vi "Read Part Details_RC.vi"(7 "Part Details in":T2, 8 "error in (no error)":errorcluster, 9 "Rack ID":u8, 10 "Part Name":string="HSG 250F (PS03)", 11 "Output Merged Cluster":variant) -> (0 "error out":errorcluster, 3 "Part Details out":T2)   [LabVIEW 2019, in "Rack Controller.lvclass"]
uses:
  Rack Controller.lvclass
  Controls/Part Details_RC.ctl
panel:
  in  "Pats List":T1
  out "Parts List":T3
  out "Error Message":string
  out "VCluster\n out":variant
  in  "Override file path":path=path "C:/Users/veenaj/Desktop/GTRON/02-11-2018/ZenGage V1.3/Configuration file/Rack Controller Parameters Override.json"
  in  "Default file path":path=path "C:/Users/veenaj/Desktop/GTRON/02-11-2018/ZenGage V1.3/Configuration file/Rack Controller Parameters Default.json"
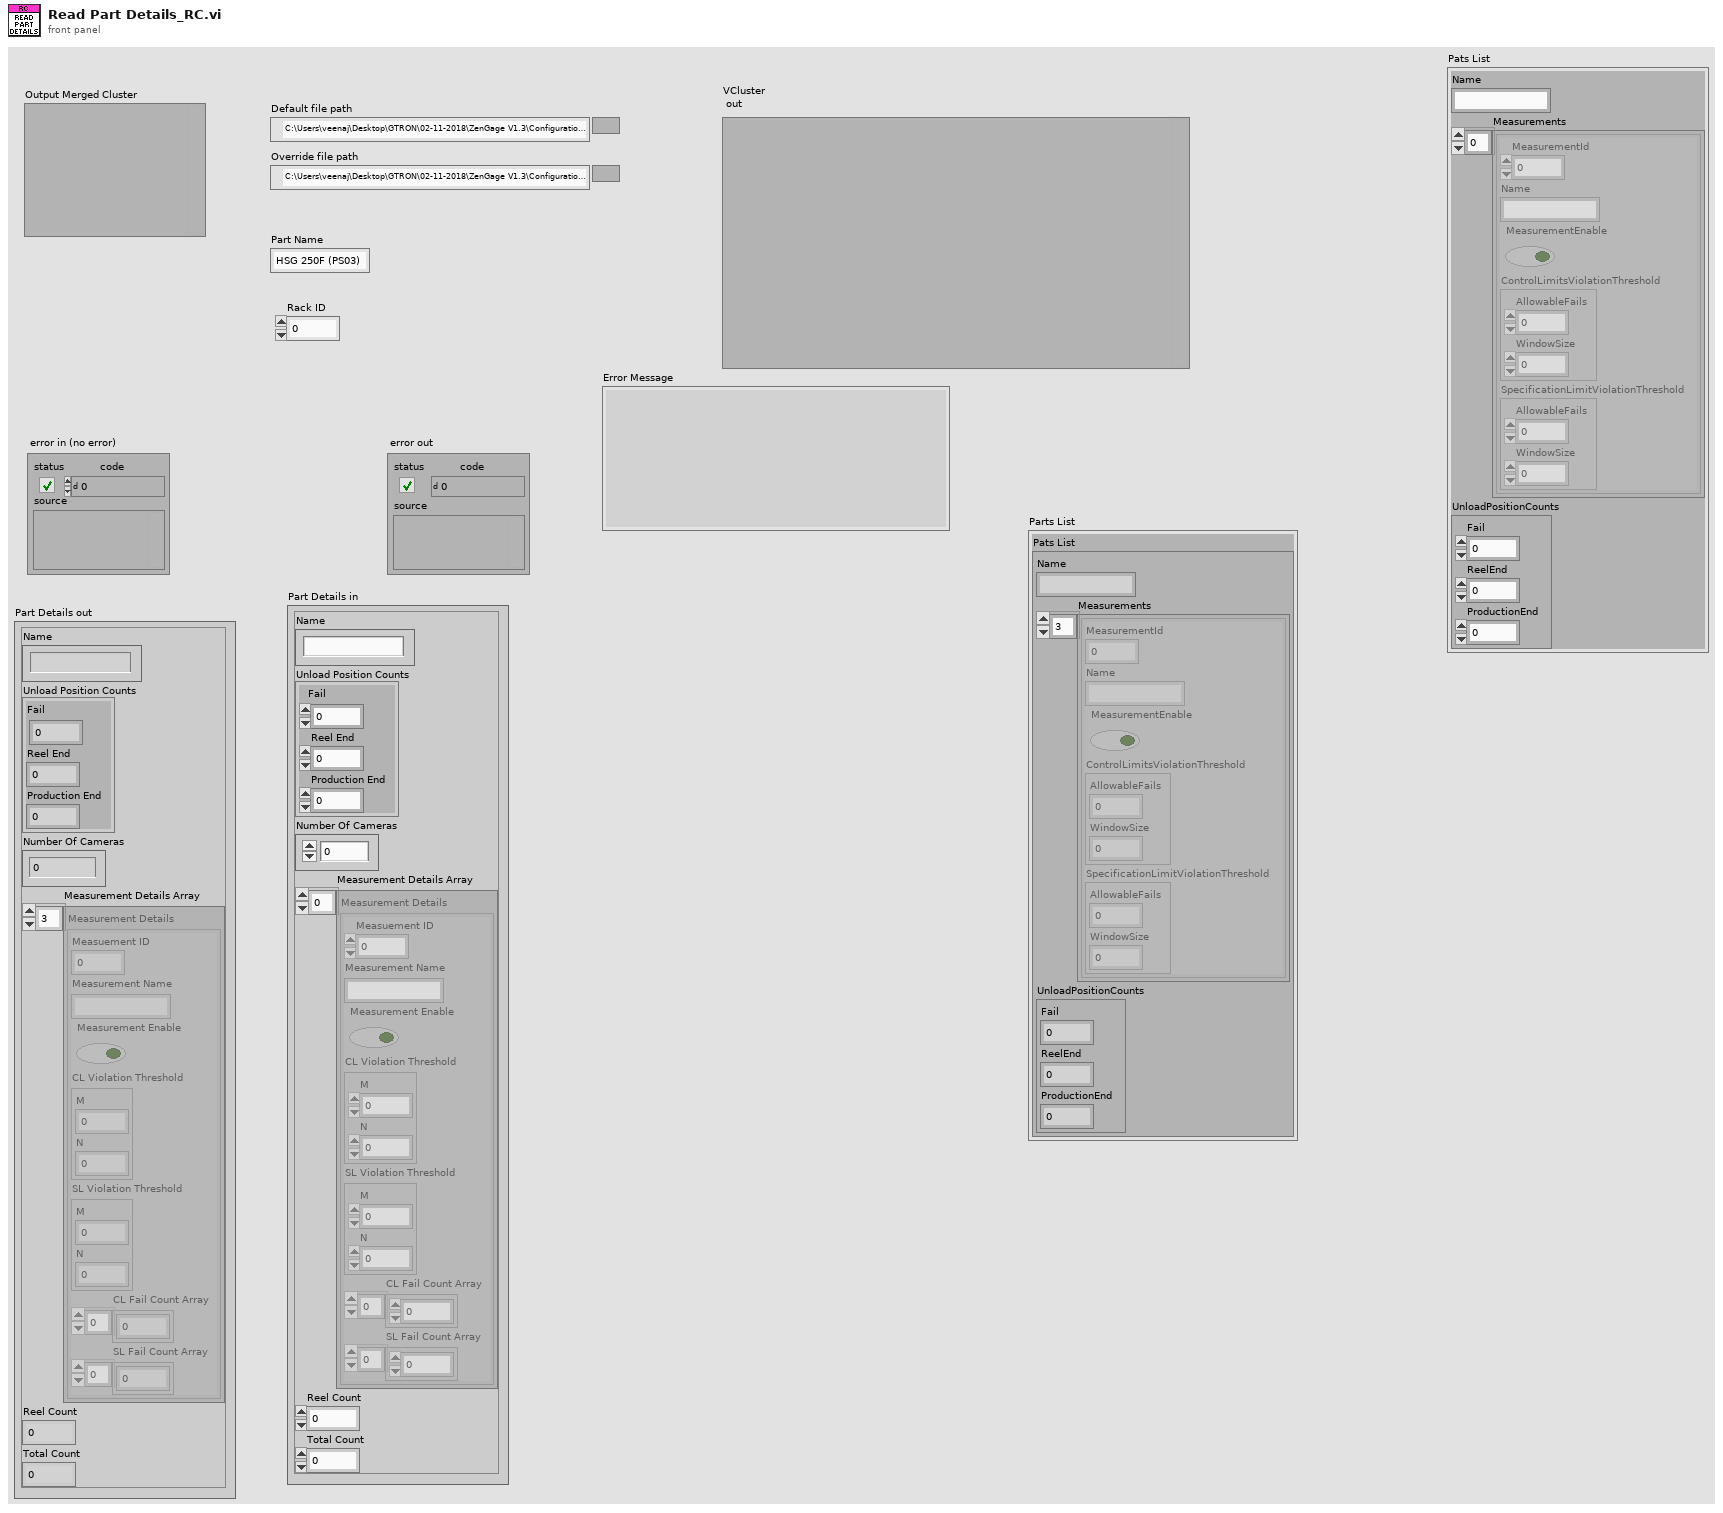
[diagram p1: front panel]
types:
  T1 = cluster{"Name":string, "Measurements":cluster{"MeasurementId":u8, "Name":string, "MeasurementEnable":bool, "ControlLimitsViolationThreshold":cluster{"AllowableFails":u64, "WindowSize":u64}, "SpecificationLimitViolationThreshold":cluster{"AllowableFails":u64, "WindowSize":u64}}[], "UnloadPositionCounts":cluster{"Fail":u64, "ReelEnd":u64, "ProductionEnd":u64}}
  T2 = typedef "Rack Controller.lvclass/Part Details_RC.ctl" = cluster{"Name":string, "Unload Position Counts":cluster{"Fail":u32, "Reel End":u32, "Production End":u32}, "Number Of Cameras":u8, "Measurement Details Array":cluster{"Measuement ID":u16, "Measurement Name":string, "Measurement Enable":bool, "CL Violation Threshold":cluster{"M":u8, "N":u64}, "SL Violation Threshold":cluster{"M":u8, "N":u64}, "CL Fail Count Array":u64[], "SL Fail Count Array":u64[]}[], "Reel Count":u64, "Total Count":u64}
  T3 = cluster{"Pats List":cluster{"Name":string, "Measurements":cluster{"MeasurementId":dbl, "Name":string, "MeasurementEnable":bool, "ControlLimitsViolationThreshold":cluster{"AllowableFails":dbl, "WindowSize":dbl}, "SpecificationLimitViolationThreshold":cluster{"AllowableFails":dbl, "WindowSize":dbl}}[], "UnloadPositionCounts":cluster{"Fail":dbl, "ReelEnd":dbl, "ProductionEnd":dbl}}}
  T4 = cluster{"Pats List":cluster{"Name":string, "Measurements":cluster{"MeasurementId":u8, "Name":string, "MeasurementEnable":bool, "ControlLimitsViolationThreshold":cluster{"AllowableFails":u64, "WindowSize":u64}, "SpecificationLimitViolationThreshold":cluster{"AllowableFails":u64, "WindowSize":u64}}[], "UnloadPositionCounts":cluster{"Fail":u64, "ReelEnd":u64, "ProductionEnd":u64}}}
  T5 = cluster{"Fail":u64, "ReelEnd":u64, "ProductionEnd":u64}
  T6 = cluster{"MeasurementId":u8, "Name":string, "MeasurementEnable":bool, "ControlLimitsViolationThreshold":cluster{"AllowableFails":u64, "WindowSize":u64}, "SpecificationLimitViolationThreshold":cluster{"AllowableFails":u64, "WindowSize":u64}}[]
  T7 = cluster{"Measuement ID":u16, "Measurement Name":string, "Measurement Enable":bool, "CL Violation Threshold":cluster{"M":u8, "N":u64}, "SL Violation Threshold":cluster{"M":u8, "N":u64}, "CL Fail Count Array":u64[], "SL Fail Count Array":u64[]}
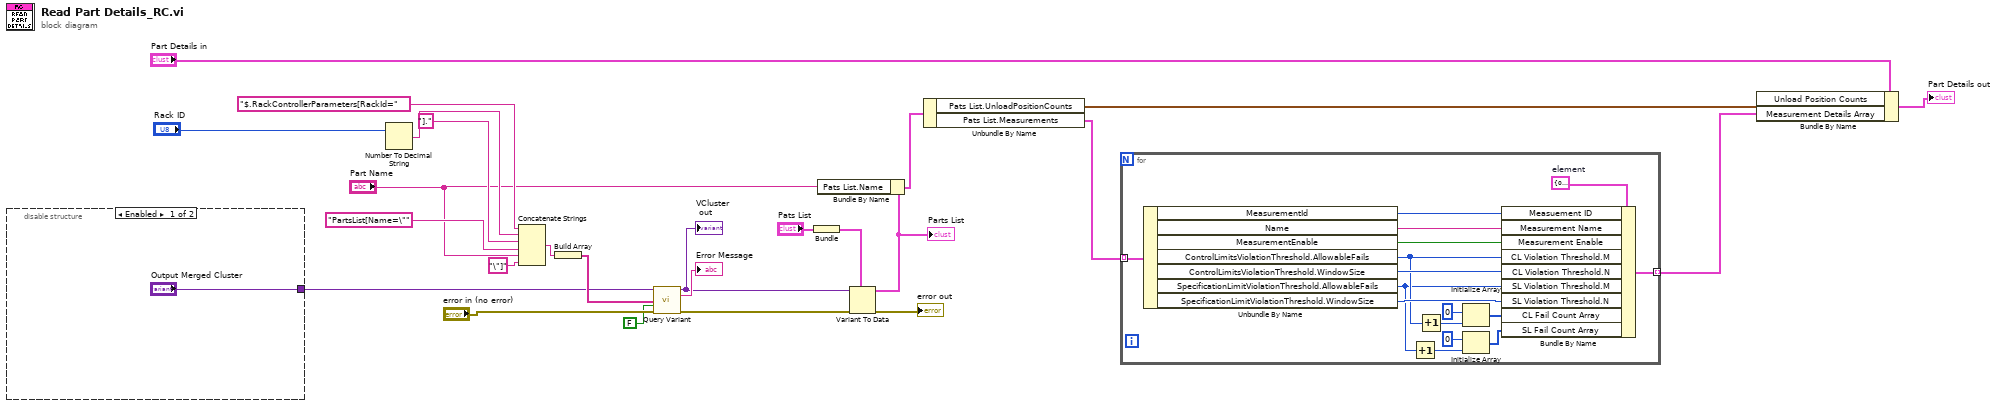
[diagram p0: block diagram]
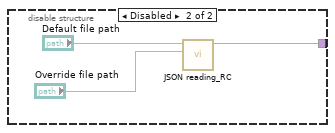
[diagram p2: hidden frame]
diagram:
  n1 = disable-structure shown="Enabled" {
    disable-tunnel: ["Output Merged Cluster" w27] -> w19
    frame Enabled {
    }
    frame Disabled {
      n2 = call "JSON reading_RC.vi"("Override file path"="Override file path", "Default file path"="Default file path") -> ("Output Merged Cluster"=w27:variant)  [unwired: 8 in, 1 out]
    }
  }
  n3 = Number To Decimal String(number="Rack ID") -> (decimal integer string=w16:string)  [unwired: 1 in]
  n4 = Concatenate Strings("$.RackControllerParameters[RackId=" ("String"), w16, "]." ("string"), "PartsList[Name=\"" ("String"), "Part Name", "\"]" ("string")) -> (w23:string)
  n5 = Build Array(w23) -> (w22:string[])
  n6 = call <vilib>:"Query Variant.vi"("VCluster in"=w19, "pathList"=w22, "Reorder\nqueried\nvariants?"=FALSE ("Reorder\nqueried\nvariants?"), "error IO"="error in (no error)") -> ("VCluster\n out"=w14:variant, "Error Message"=→"Error Message":string, "error out"=w13:errorcluster)  [unwired: 8 in, 1 out]
  "VCluster\n out" <- w14
  n7 = Bundle("Pats List"="Pats List") -> (w10:T4)  [unwired: 1 in]
  n8 = Variant To Data(error in=w13, type=w10, Variant=w14) -> (data=w4:T4, error out=→"error out":errorcluster)
  "Parts List" <- w4
  n9 = Bundle By Name(cluster=w4, "Pats List.Name"="Part Name") -> (w3:T4)
  n10 = Unbundle By Name(w3) -> ("Pats List.UnloadPositionCounts"=w8:T5, "Pats List.Measurements"=w9:T6)
  n11 = for {
    tunnel: w9 -> [w45] mode=indexing
    tunnel: [w34] -> w5 mode=indexing
    w35 = T7 {"Measuement ID"=0, "Measurement Name"="", "Measurement Enable"=FALSE, "CL Violation Threshold"={"M"=0, "N"=0}, "SL Violation Threshold"={"M"=0, "N"=0}, "CL Fail Count Array"=[], "SL Fail Count Array"=[]}  # element
    n12 = Unbundle By Name(w45) -> ("MeasurementId"=w44:u8, "Name"=w43:string, "MeasurementEnable"=w36:bool, "ControlLimitsViolationThreshold.AllowableFails"=w33:u64, "ControlLimitsViolationThreshold.WindowSize"=w40:u64, "SpecificationLimitViolationThreshold.AllowableFails"=w32:u64, "SpecificationLimitViolationThreshold.WindowSize"=w39:u64)
    n13 = Increment(x=w32) -> (x+1=w30:u64)
    n14 = Increment(x=w33) -> (x+1=w31:u64)
    n15 = Initialize Array(u64 0, w31) -> (w38:u64[])
    n16 = Initialize Array(u64 0, w30) -> (w37:u64[])
    n17 = Bundle By Name(cluster=w35, "Measuement ID"=w44, "Measurement Name"=w43, "Measurement Enable"=w36, "CL Violation Threshold.M"=w33, "CL Violation Threshold.N"=w40, "SL Violation Threshold.M"=w32, "SL Violation Threshold.N"=w39, "CL Fail Count Array"=w38, "SL Fail Count Array"=w37) -> (w34:T7)
  }
  n18 = Bundle By Name(cluster="Part Details in", "Unload Position Counts"=w8, "Measurement Details Array"=w5) -> (→"Part Details out":T2)
